vi "Dual Channel Log with Prompt Cancellation Handling.vi"() -> ()   [LabVIEW 2014]
doc: "本VI每间隔1秒采集温度值，并持续计算最近5次温度值的平均值。本VI显示并计算原始数据和实时平均值。"
uses:
  File Operation.ctl
panel:
  in  "停止按钮":bool
  out "温度历史":cluster{dbl, "Temperature Value":dbl}(graph)
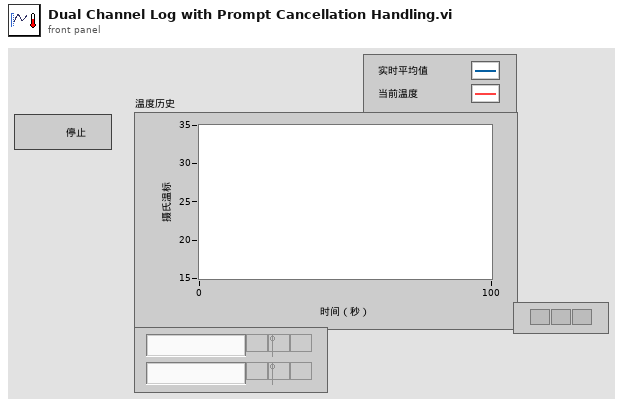
[diagram p1: front panel]
types:
  T1 = enum16{"open", "replace", "create", "open or create", "replace or create", "replace or create with confirmation"}
  T2 = typedef "File Operation.ctl" = enum16{"提示用户", "写入数据", "禁止写入"}
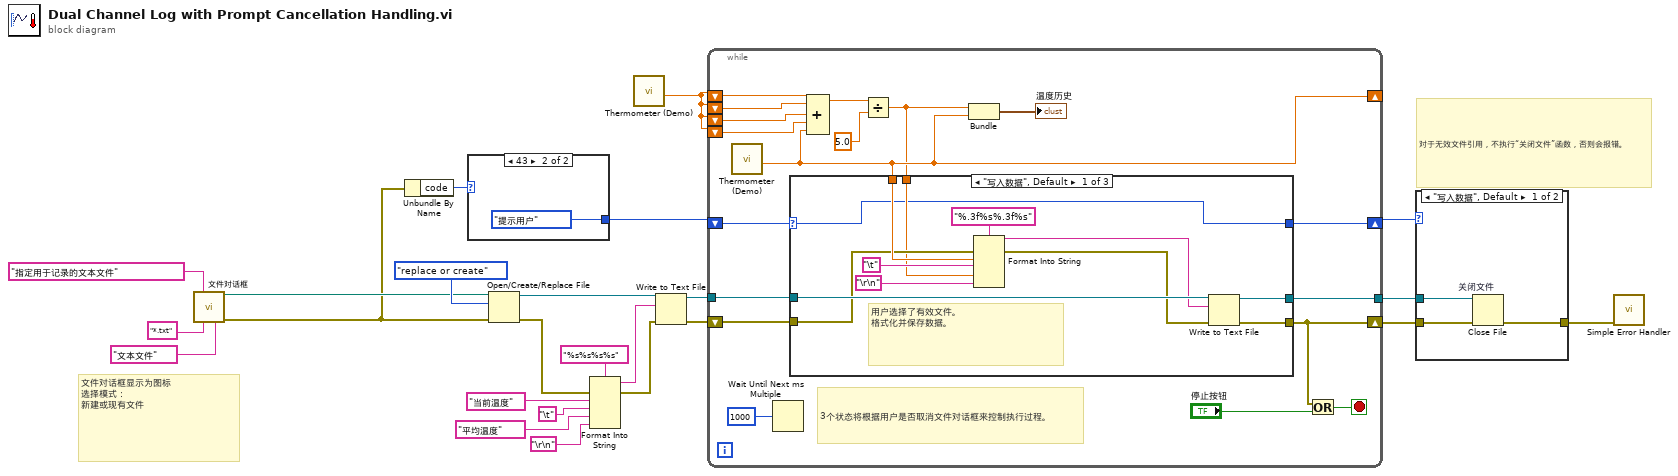
[diagram p0: block diagram]
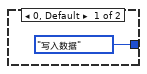
[diagram p3: hidden frame]
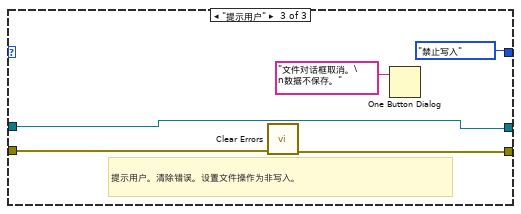
[diagram p5: hidden frame]
diagram:
  # "对于无效文件引用，不执行“关闭文件”函数，否则会报错。"
  # "文件对话框显示为图标\n选择模式：\n新建或现有文件"
  n1 = call "文件对话框"("prompt"="指定用于记录的文本文件" ("类型标签"), "pattern (all files)"="*.txt" ("类型（所有文件）"), "pattern label"="文本文件" ("类型标签")) -> ("selected path"=w18:path, "error out"=w4:errorcluster)  [unwired: 9 in, 2 out]
  n2 = Unbundle By Name(w4) -> ("code"=w5:i32)
  n3 = case shown="43" w5 {
    tunnel: [File_Operation."写入数据" ("枚举") File_Operation."提示用户" ("枚举")] -> w3
    frame 0, Default {
    }
    frame 43 {
    }
  }
  n4 = Open/Create/Replace File(file path (use dialog)=w18, error in=w4, operation (0:open)=T1."replace or create" ("操作(0:open)")) -> (refnum out=w19:refnum<file>, error out=w7:errorcluster)  [unwired: 4 out]
  n5 = Format Into String(format string="%s%s%s%s" ("格式字符串"), error in=w7, "当前温度" ("字符串"), "\t" ("制表符常量"), "平均温度" ("字符串"), "\r\n" ("行结束常量")) -> (resulting string=w8:string, error out=w6:errorcluster)  [unwired: 1 in]
  n6 = call "Thermometer (Demo).vi"() -> ("温度值"=w24:dbl)  [unwired: 11 in]
  n7 = Write to Text File(file (use dialog)=w19, text=w8, error in=w6) -> (refnum out=w15:refnum<file>, error out=w14:errorcluster)  [unwired: 2 out]
  n8 = while {
    shift-right: [w31] -> _
    shift-left: w24 -> [w43]
    shift-left: w24 -> [w42]
    shift-left: w24 -> [w39]
    shift-left: w24 -> [w38]
    tunnel: w15 -> [w36]
    tunnel: [w35] -> w21
    shift-right: [w27] -> w2
    shift-left: w3 -> [w28]
    shift-right: [w34] -> w22
    shift-left: w14 -> [w30]
    stop <- w32 stop-if-true
    # "3个状态将根据用户是否取消文件对话框来控制执行过程。"
    n9 = call "Thermometer (Demo).vi"() -> ("温度值"=w31:dbl)  [unwired: 11 in]
    n10 = Wait Until Next ms Multiple(millisecond multiple=u32 1000 ("毫秒倍数")) -> ()  [unwired: 1 out]
    n11 = Compound Arithmetic op=ADD(w43, w42, w39, w38, w31) -> (w41:dbl)
    n12 = Divide(x=w41, y=5.0) -> (x/y=w29:dbl)
    n13 = case shown="\"写入数据\", Default" w28 {
      selector: w28 -> [w45 w59 _]
      tunnel: w36 -> [w56 w58 w61]
      tunnel: [w55 w58 w61] -> w35
      tunnel: [w54 w57 w62] -> w34
      tunnel: w31 -> [w53 _ _]
      tunnel: w30 -> [w51 w57 w63]
      tunnel: w29 -> [w46 _ _]
      tunnel: [w45 w59 File_Operation."禁止写入" ("枚举")] -> w27
      frame "写入数据", Default {
        # "用户选择了有效文件。\n格式化并保存数据。"
        n14 = Format Into String(format string="%.3f%s%.3f%s" ("格式字符串"), error in=w51, w53, "\t" ("制表符常量"), w46, "\r\n" ("行结束常量")) -> (resulting string=w52:string, error out=w50:errorcluster)  [unwired: 1 in]
        n15 = Write to Text File(file (use dialog)=w56, text=w52, error in=w50) -> (refnum out=w55:refnum<file>, error out=w54:errorcluster)  [unwired: 2 out]
      }
      frame "禁止写入" {
        # "退出程序，不要保存数据。"
      }
      frame "提示用户" {
        # "提示用户。清除错误。设置文件操作为非写入。"
        n16 = call <vilib>:"Clear Errors.vi"("error in (no error)"=w63) -> ("error out"=w62:errorcluster)  [unwired: 5 in, 1 out]
        n17 = One Button Dialog(message="文件对话框取消。\n数据不保存。" ("消息")) -> ()  [unwired: 1 in, 1 out]
      }
    }
    n18 = Bundle(w29, "温度值"=w31) -> (→"温度历史":cluster{dbl, "温度值":dbl})  [unwired: 1 in]
    n19 = Or(x=w34, y="停止按钮") -> (x .or. y?=w32:bool)
  }
  n20 = case shown="\"写入数据\", Default" w2 {
    tunnel: [w67 w68] -> w23
    tunnel: w22 -> [w66 w68]
    tunnel: w21 -> [w65 _]
    frame "写入数据", Default {
      n21 = Close File "关闭文件"(refnum=w65, error in=w66) -> (error out=w67:errorcluster)  [unwired: 1 out]
    }
    frame "禁止写入" {
    }
  }
  n22 = call <vilib>:"Simple Error Handler.vi"("error in (no error)"=w23) -> ()  [unwired: 1 in, 8 out]
